vi "..face set up.vi"() -> ()   [LabVIEW 2018]
doc: "This example shows how to capture and display an image from a grab acquisition\n\nSteps to run:\n\n1. Ensure interface name is correct for your camera and system setup\n2. Run the VI\n3. When you want to capture an image click the Get Image control."
uses:
  <vilib>/vision/Image Controls.llb/IMAQ Image.ctl
  <vilib>/University of Leeds/Kinesthesia Toolkit for Microsoft Kinect/_Polymorphic Configure/Event-Video.vi
  <vilib>/University of Leeds/Kinesthesia Toolkit for Microsoft Kinect/_Polymorphic Read/Read-Video.vi
  <vilib>/University of Leeds/Kinesthesia Toolkit for Microsoft Kinect/_Polymorphic Close/Close-Video.vi
panel:
  in  "stop":bool
  out "RGB":T1
  out "new picture":picture
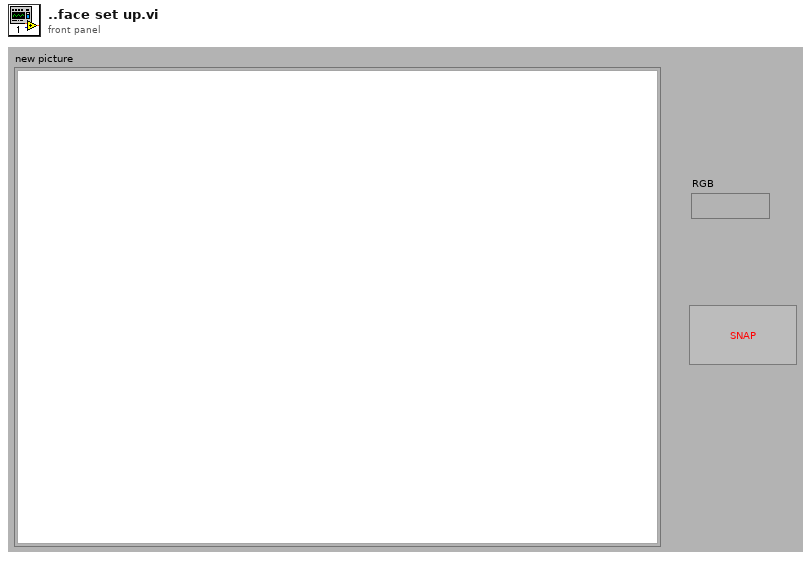
[diagram p1: front panel]
types:
  T1 = typedef "IMAQ Image.ctl" = refnum<image>
  T2 = typedef "Image Type" = u32
  T3 = cluster{cluster{"reference out":refnum<k24>, "KinectSensors":refnum<k24>}, "get_Item":refnum<k24>}
  T4 = cluster{"reference out":refnum<k24>, "KinectSensors":refnum<k24>, "ColorStream":refnum<k24>, "get_Item":refnum<k24>}
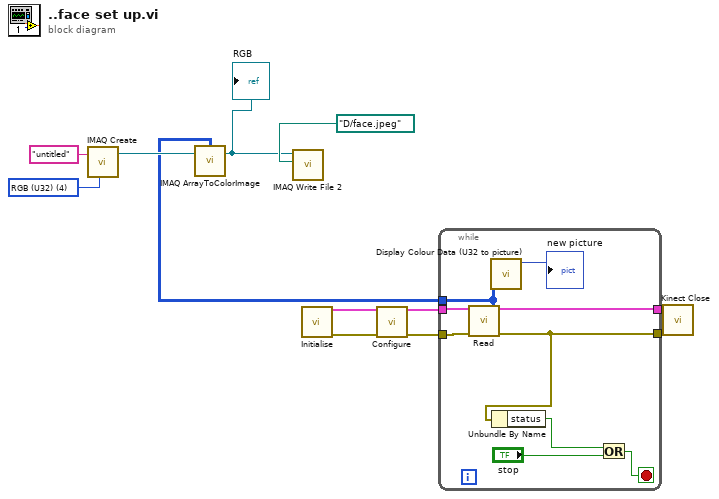
[diagram p0: block diagram]
diagram:
  w6 = T2 4 items=["Grayscale (U8)", "Grayscale (I16)", "Grayscale (SGL)", "Complex (CSG)", "RGB (U32)", "HSL (U32)", "RGB (U64)", "Grayscale (U16)"] ("Image Type")
  n1 = call "IMAQ Create"("Image Name"="untitled", "Image Type"=w6) -> ("New Image"=w8:T1)  [unwired: 3 in, 1 out]
  n2 = call <vilib>:"Initialise.vi"() -> ("Kinect References out"=w10:T3, "error out"=w11:errorcluster)  [unwired: 14 in]
  n3 = call-poly <vilib>:"Configure.vi"("Kinect References in"=w10, "error in"=w11) -> ("Kinect References out"=w9:T4, "error out"=w3:errorcluster)  [unwired: 12 in]
  n4 = while {
    tunnel: [w21] -> w12
    tunnel: w9 -> [w20]
    tunnel: [w19] -> w5
    tunnel: w3 -> [w17]
    tunnel: [w14] -> w1
    stop <- w13 stop-if-true
    n5 = call-poly <vilib>:"Read.vi"("Kinect References in"=w20, "error in (no error)"=w17) -> ("Colour output array (U24, RGB)"=w19:u32[][], "Kinect References out"=w21:T4, "error out"=w14:errorcluster)  [unwired: 10 in, 1 out]
    n6 = call <vilib>:"Display Colour Data (U32 to picture).vi"("Colour output array (U24, RGB)"=w19) -> ("new picture"=→"new picture":picture)  [unwired: 10 in]
    n7 = Unbundle By Name(w14) -> ("status"=w16:bool)
    n8 = Or(x=w16, y="stop") -> (x .or. y?=w13:bool)
  }
  n9 = call "IMAQ ArrayToColorImage"("Image Pixels (U32)"=w5, "Image"=w8) -> ("Image Out"=w2:T1)  [unwired: 3 in, 1 out]
  "RGB" <- w2
  n10 = call-poly "IMAQ Write File 2"("File Path"=path "D:/face.jpeg", "Image"=w2) -> ()  [unwired: 8 in, 2 out]
  n11 = call-poly <vilib>:"Kinect Close.vi"("Kinect References in"=w12, "error in"=w1) -> ()  [unwired: 13 in, 1 out]
